vi "1D Array (Range[0,N-1]).vi"(2 "Range":i32) -> (16 "Array":i32[](array[numeric]))   [LabVIEW 2014]
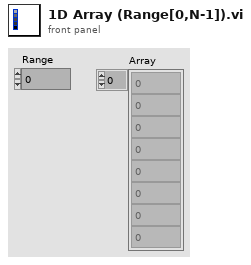
[diagram p1: front panel]
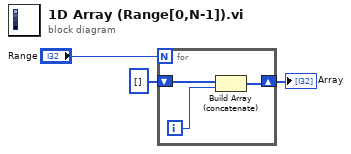
[diagram p0: block diagram]
diagram:
  n1 = for {
    N: "Range" -> [_]
    shift-right: [w5] -> w1
    shift-left: i32[] [] -> [w4]
    i -> [w6]
    n2 = Build Array (concatenate)(w4, w6) -> (w5:i32[])
  }
  "Array" <- w1
